vi "RC_Client 3.vi"() -> ()   [LabVIEW 2019, in "RemoteControl.lvclass"]
uses:
  RemoteControl/RemoteControl.lvclass
  RemoteControl.STM.lvclass
  C:/user/patrick/git/LevyLab-Instrument-Framework/lvsrc/SMOs/RemoteControl/RemoteControl.lvclass
  RemoteControl.ZMQ/RemoteControl.ZMQ.lvclass
  <userlib>/_OpenG.lib/numeric/numeric.llb/Random Number Within Range - I32__ogtk.vi
  <userlib>/_OpenG.lib/error/error.llb/Filter Error Codes (Array)__ogtk.vi
panel:
  in  "Type":enum16{"RC", "STM", "ZMQ"}(ring)=enum."ZMQ"
  in  "milliseconds to wait":u32
  out "time (1 message) (ms)":u32
  out "startup time (ms)":u32
  out "messsages/s":dbl
  in  "remote port":u16=6341
  in  "address":string
  out "Data":variant
  out "Messages":i32
  in  "Stop":bool
  out "Command reponse":string
  out "Command":string
  out "meta data\n(available commands)":string
  out "error out":errorcluster
  # "CLIENT (API)"
  # "Connection info"
  # "Message Sent"
  # "Message Received"
  # "Metrics"
  # "3"
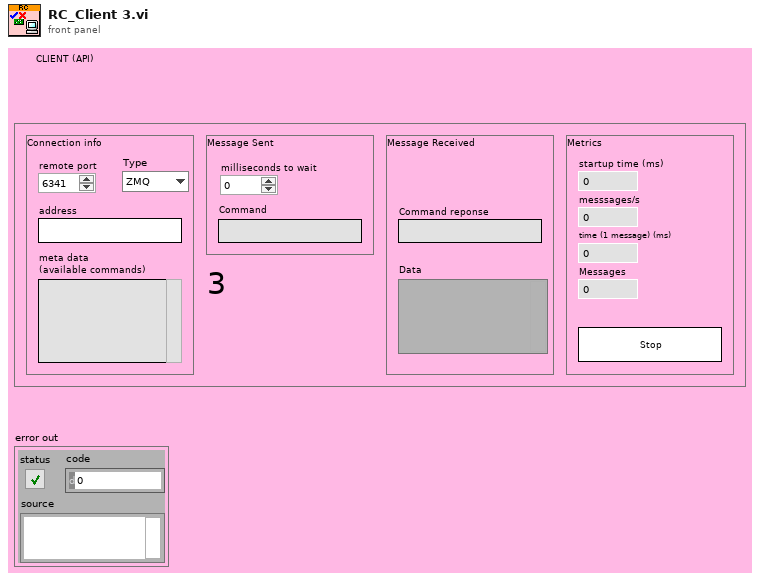
[diagram p1: front panel]
types:
  T1 = cluster{"Command out":string, "Data out":variant, i32}
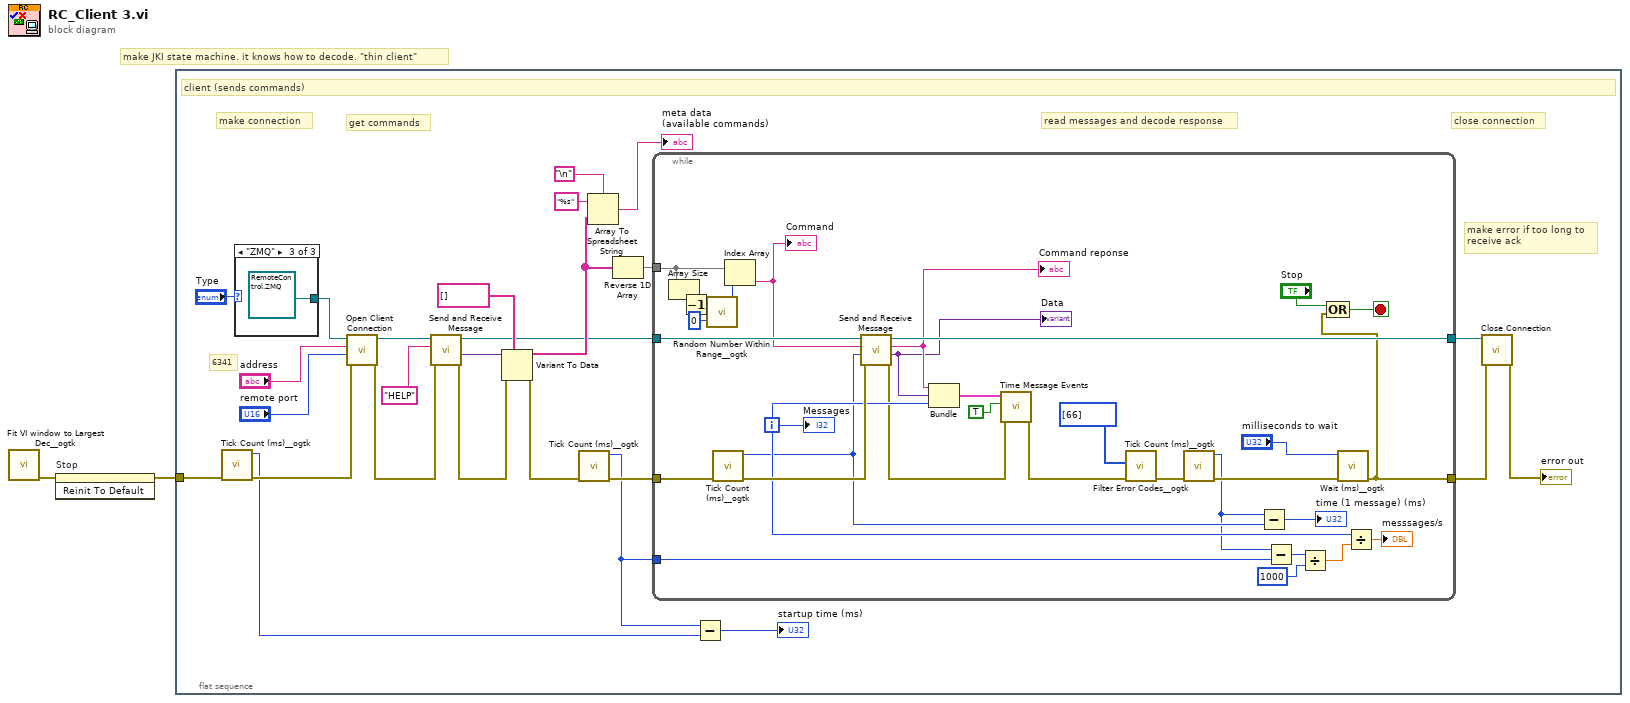
[diagram p0: block diagram]
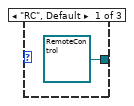
[diagram p2: hidden frame]
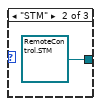
[diagram p3: hidden frame]
diagram:
  # "make JKI state machine. it knows how to decode. \"thin client\""
  n1 = call <userlib>:"Fit VI window to Largest Dec__ogtk.vi"() -> ("error out"=w2:errorcluster)  [unwired: 6 in, 1 out]
  n2 = invoke on="Stop" class="Bool" method="Reinit To Default"(error in=w2) -> (error out=w1:errorcluster)  [unwired: 2 in, 2 out]
  n3 = flat-sequence {
    tunnel: w1 -> [w12]
    frame #0 {
      # "close connection"
      # "read messages and decode response"
      # "get commands"
      # "make connection"
      # "6341"
      # "make error if too long to\nreceive ack"
      # "client (sends commands)"
      n4 = call <userlib>:"Tick Count (ms)__ogtk.vi"("error in (no error)"=w12) -> ("error out"=w23:errorcluster, "millisecond timer value"=w20:u32)  [unwired: 9 in]
      n5 = case shown="\"ZMQ\"" "Type" {
        tunnel: [refnum<class "RemoteControl.lvclass"> refnum ("SMO.Template.lvclass") refnum<class "RemoteControl.STM.lvclass"> refnum ("RemoteControl.STM.lvclass") refnum<class "RemoteControl.ZMQ.lvclass"> refnum ("RemoteControl.ZMQ.lvclass")] -> w13
        frame "RC", Default {
        }
        frame "STM" {
        }
        frame "ZMQ" {
        }
      }
      n6 = call-dynamic "Open Client Connection.vi"("error in (no error)"=w23, "Port"="remote port", "address"="address", "RemoteControl in"=w13) -> ("error out"=w11:errorcluster, "RemoteControl out"=w9:refnum<class "RemoteControl.lvclass">)  [unwired: 6 in]
      n7 = call-dynamic "Send and Receive Message.vi"("error in (no error)"=w11, "Command"="HELP", "RemoteControl in"=w9) -> ("error out"=w5:errorcluster, "Data out"=w7:variant, "RemoteControl out"=w3:refnum<class "RemoteControl.lvclass">)  [unwired: 5 in, 1 out]
      n8 = Variant To Data(error in=w5, type=string[] [], Variant=w7) -> (data=w8:string[], error out=w4:errorcluster)
      n9 = call <userlib>:"Tick Count (ms)__ogtk.vi"("error in (no error)"=w4) -> ("error out"=w22:errorcluster, "millisecond timer value"=w15:u32)  [unwired: 9 in]
      n10 = Array To Spreadsheet String(delimiter (Tab)="\n", array=w8, 3:"%s" ("format string")) -> (spreadsheet string=→"meta data\n(available commands)":string)
      n11 = Reverse 1D Array(array=w8) -> (reversed array=w24:string[])
      n12 = while {
        tunnel: [w40] -> w28
        tunnel: [w60] -> w27
        tunnel: w22 -> [w55]
        tunnel: w3 -> [w61]
        tunnel: w24 -> [w44]
        tunnel: w15 -> [w34]
        i -> [w52]
        stop <- w63 stop-if-true
        n13 = Array Size(array=w44) -> (size(s)=w45:i32)
        n14 = Decrement(x=w45) -> (x-1=w43:i32)
        n15 = call-poly <userlib>:"Random Number Within Range__ogtk.vi"("High"=w43, "Low"=0) -> ("Random Number"=w47:i32)  [unwired: 3 in]
        n16 = call <userlib>:"Tick Count (ms)__ogtk.vi"("error in (no error)"=w55) -> ("error out"=w54:errorcluster, "millisecond timer value"=w41:u32)  [unwired: 9 in]
        n17 = Index Array(array=w44, index=w47) -> (element=w56:string)
        "Command" <- w56
        n18 = call-dynamic "Send and Receive Message.vi"("error in (no error)"=w54, "Data"=w41, "Command"=w56, "RemoteControl in"=w61) -> ("error out"=w42:errorcluster, "Data out"=w32:variant, "Command out"=w53:string, "RemoteControl out"=w60:refnum<class "RemoteControl.lvclass">)  [unwired: 4 in]
        "Command reponse" <- w53
        "Data" <- w32
        n19 = Bundle("Command out"=w53, "Data out"=w32, w52) -> (w51:T1)  [unwired: 1 in]
        n20 = call "Time Message Events.vi"("error in (no error)"=w42, "Debug Mode"=TRUE, "Message in"=w51) -> ("error out"=w33:errorcluster)  [unwired: 6 in, 2 out]
        n21 = call-poly <userlib>:"Filter Error Codes__ogtk.vi"("Error In"=w33, "Error Codes to Filter"=i32[] [66]) -> ("Error Out"=w59:errorcluster)  [unwired: 7 in, 2 out]
        n22 = call <userlib>:"Tick Count (ms)__ogtk.vi"("error in (no error)"=w59) -> ("error out"=w49:errorcluster, "millisecond timer value"=w36:u32)  [unwired: 9 in]
        n23 = Subtract(x=w36, y=w41) -> (x-y=→"time (1 message) (ms)":u32)
        n24 = Subtract(x=w36, y=w34) -> (x-y=w35:u32)
        n25 = Divide(x=w35, y=u32 1000) -> (x/y=w58:dbl)
        n26 = call <userlib>:"Wait (ms)__ogtk.vi"("error in (no error)"=w49, "milliseconds to wait"="milliseconds to wait") -> ("error out"=w40:errorcluster)  [unwired: 8 in, 1 out]
        n27 = Compound Arithmetic op=OR("Stop", w40) -> (w63:bool)
        n28 = Divide(x=w52, y=w58) -> (x/y=→"messsages/s":dbl)
        "Messages" <- w52
      }
      n29 = Subtract(x=w15, y=w20) -> (x-y=→"startup time (ms)":u32)
      n30 = call-dynamic "Close Connection.vi"("error in (no error)"=w28, "RemoteControl in"=w27) -> ("error out"=→"error out":errorcluster)  [unwired: 8 in, 1 out]
    }
  }
